vi "UpdateLogStrings.vi"(8 "error in (no error)":errorcluster, 11 "object in":refnum<class "EventLogger_Actor.lvclass">) -> (0 "error out":errorcluster, 3 "object out":refnum<class "EventLogger_Actor.lvclass">)   [LabVIEW 2014, in "EventLogger_Actor.lvlib" / "EventLogger_Actor.lvclass"]
uses:
  EventLogger_Actor.lvclass
  EventLogger_Actor.lvclass/EventLogger_Actor.ctl
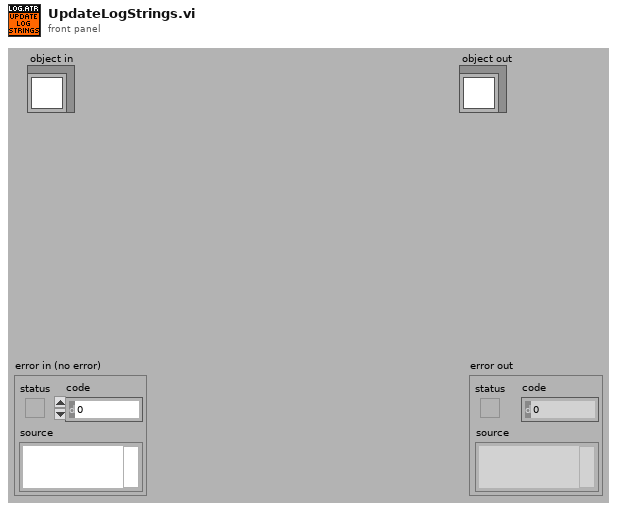
[diagram p1: front panel]
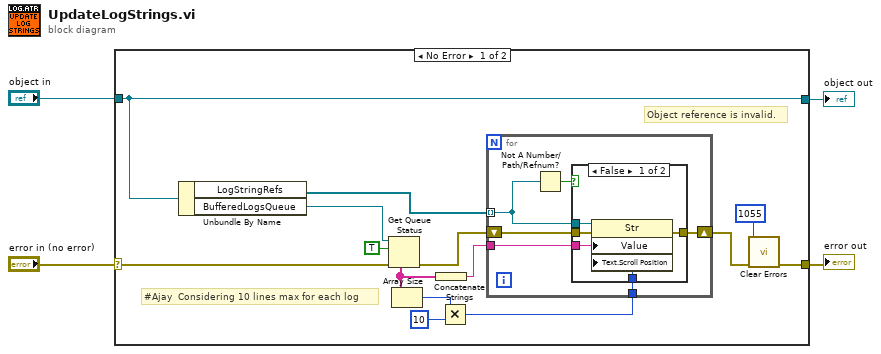
[diagram p0: block diagram]
diagram:
  n1 = case shown="No Error" "error in (no error)" {
    selector: "error in (no error)" -> [w18 w32]
    tunnel: [w6 w32] -> w3
    tunnel: [w17 w31] -> w1
    tunnel: "object in" -> [w17 w31]
    frame No Error {
      # "Object reference is invalid."
      # "#Ajay  Considering 10 lines max for each log"
      n2 = Unbundle By Name(w17) -> ("LogStringRefs"=w14:refnum<vi>[], "BufferedLogsQueue"=w16:refnum<queue>)
      n3 = Get Queue Status(queue=w16, return elements? (F)=TRUE, error in (no error)=w18) -> (error out=w12:errorcluster, elements=w10:string[])  [unwired: 6 out]
      n4 = Array Size(array=w10) -> (size(s)=w9:i32)
      n5 = Concatenate Strings(w10) -> (w11:string)
      n6 = Multiply(x=w9, y=10) -> (x*y=w7:i32)
      n7 = for {
        tunnel: w14 -> [w20] mode=indexing
        shift-right: [w23] -> w13
        shift-left: w12 -> [w24]
        tunnel: w11 -> [w22]
        tunnel: w7 -> [w21]
        n8 = Not A Number/Path/Refnum?(number/path/refnum=w20) -> (NaN/Path/Refnum?=w19:bool)
        n9 = case shown="False" w19 {
          tunnel: w24 -> [w29 w30]
          tunnel: [w28 w30] -> w23
          tunnel: w22 -> [w27 _]
          tunnel: w21 -> [w26 _]
          tunnel: w20 -> [w25 _]
          frame False {
            n10 = property class="Str"(reference=w25, error in=w29, "Value"=w27, "Text.Scroll Position"=w26) -> (error out=w28:errorcluster)  [unwired: 1 out]
          }
          frame True {
          }
        }
      }
      n11 = call <vilib>:"Clear Errors.vi"("error in (no error)"=w13, "specific error code to clear (0: all)"=1055) -> ("error out"=w6:errorcluster)  [unwired: 4 in, 1 out]
    }
    frame Error {
    }
  }
  "error out" <- w3
  "object out" <- w1
